vi "WLAN_FrameSync - Optimized.vi"(11 "input cluster":cluster{"t0":dbl, "dt":dbl, "Y":cdb[]}) -> (2 "is valid packet?":bool, 3 "output cluster":cluster{"t0":dbl, "dt":dbl, "Y":cdb[]})   [LabVIEW 2022 SP3]
uses:
  <vilib>/Analysis/2dsp.llb/1D Cross Correlation (CDB).vi
  <vilib>/Analysis/NI_AALPro.lvlib
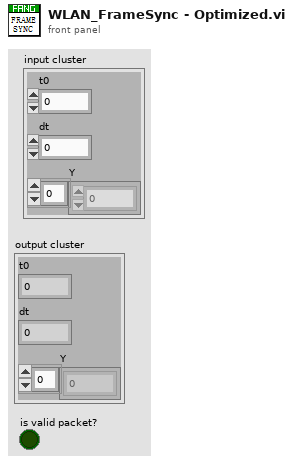
[diagram p1: front panel]
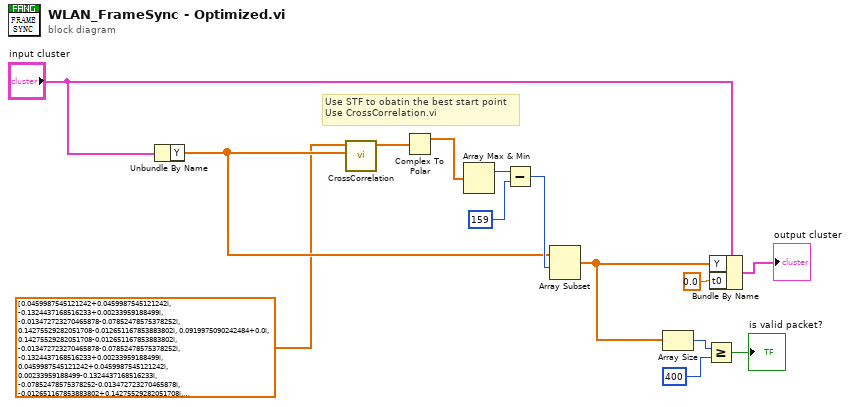
[diagram p0: block diagram]
diagram:
  # "Use STF to obatin the best start point\nUse CrossCorrelation.vi"
  n1 = Unbundle By Name("input cluster") -> ("Y"=w2:cdb[])
  n2 = call-poly <vilib>:"CrossCorrelation.vi"("Y"=w2, "X"=cdb[] [0.0459987545121242+0.0459987545121242i, -0.1324437168516233+0.00233959188499i, -0.013472723270465878-0.07852478575378252i, 0.14275529282051708-0.012651167853883802i, 0.0919975090242484+0.0i, 0.14275529282051708-0.012651167853883802i, -0.013472723270465878-0.07852478575378252i, -0.1324437168516233+0.00233959188499i, 0.0459987545121242+0.0459987545121242i, 0.00233959188499-0.1324437168516233i, -0.07852478575378252-0.013472723270465878i, -0.012651167853883802+0.14275529282051708i, 0.0+0.0919975090242484i, -0.012651167853883802+0.14275529282051708i, -0.07852478575378252-0.013472723270465878i, 0.00233959188499-0.1324437168516233i, 0.0459987545121242+0.0459987545121242i, -0.1324437168516233+0.00233959188499i, -0.013472723270465878-0.07852478575378252i, 0.14275529282051708-0.012651167853883802i, 0.0919975090242484+0.0i, 0.14275529282051708-0.012651167853883802i, -0.013472723270465878-0.07852478575378252i, -0.1324437168516233+0.00233959188499i, 0.0459987545121242+0.0459987545121242i, 0.00233959188499-0.1324437168516233i, -0.07852478575378252-0.013472723270465878i, -0.012651167853883802+0.14275529282051708i, 0.0+0.0919975090242484i, -0.012651167853883802+0.14275529282051708i, -0.07852478575378252-0.013472723270465878i, 0.00233959188499-0.1324437168516233i, 0.0459987545121242+0.0459987545121242i, -0.1324437168516233+0.00233959188499i, -0.013472723270465878-0.07852478575378252i, 0.14275529282051708-0.012651167853883802i, 0.0919975090242484+0.0i, 0.14275529282051708-0.012651167853883802i, -0.013472723270465878-0.07852478575378252i, -0.1324437168516233+0.00233959188499i, 0.0459987545121242+0.0459987545121242i, 0.00233959188499-0.1324437168516233i, -0.07852478575378252-0.013472723270465878i, -0.012651167853883802+0.14275529282051708i, 0.0+0.0919975090242484i, -0.012651167853883802+0.14275529282051708i, -0.07852478575378252-0.013472723270465878i, 0.00233959188499-0.1324437168516233i, 0.0459987545121242+0.0459987545121242i, -0.1324437168516233+0.00233959188499i, -0.013472723270465878-0.07852478575378252i, 0.14275529282051708-0.012651167853883802i, 0.0919975090242484+0.0i, 0.14275529282051708-0.012651167853883802i, -0.013472723270465878-0.07852478575378252i, -0.1324437168516233+0.00233959188499i, 0.0459987545121242+0.0459987545121242i, 0.00233959188499-0.1324437168516233i, -0.07852478575378252-0.013472723270465878i, -0.012651167853883802+0.14275529282051708i, 0.0+0.0919975090242484i, -0.012651167853883802+0.14275529282051708i, -0.07852478575378252-0.013472723270465878i, 0.00233959188499-0.1324437168516233i, 0.0459987545121242+0.0459987545121242i, -0.1324437168516233+0.00233959188499i, -0.013472723270465878-0.07852478575378252i, 0.14275529282051708-0.012651167853883802i, 0.0919975090242484+0.0i, 0.14275529282051708-0.012651167853883802i, -0.013472723270465878-0.07852478575378252i, -0.1324437168516233+0.00233959188499i, 0.0459987545121242+0.0459987545121242i, 0.00233959188499-0.1324437168516233i, -0.07852478575378252-0.013472723270465878i, -0.012651167853883802+0.14275529282051708i, 0.0+0.0919975090242484i, -0.012651167853883802+0.14275529282051708i, -0.07852478575378252-0.013472723270465878i, 0.00233959188499-0.1324437168516233i, 0.0459987545121242+0.0459987545121242i, -0.1324437168516233+0.00233959188499i, -0.013472723270465878-0.07852478575378252i, 0.14275529282051708-0.012651167853883802i, 0.0919975090242484+0.0i, 0.14275529282051708-0.012651167853883802i, -0.013472723270465878-0.07852478575378252i, -0.1324437168516233+0.00233959188499i, 0.0459987545121242+0.0459987545121242i, 0.00233959188499-0.1324437168516233i, -0.07852478575378252-0.013472723270465878i, -0.012651167853883802+0.14275529282051708i, 0.0+0.0919975090242484i, -0.012651167853883802+0.14275529282051708i, -0.07852478575378252-0.013472723270465878i, 0.00233959188499-0.1324437168516233i, 0.0459987545121242+0.0459987545121242i, -0.1324437168516233+0.00233959188499i, -0.013472723270465878-0.07852478575378252i, 0.14275529282051708-0.012651167853883802i, 0.0919975090242484+0.0i, 0.14275529282051708-0.012651167853883802i, -0.013472723270465878-0.07852478575378252i, -0.1324437168516233+0.00233959188499i, 0.0459987545121242+0.0459987545121242i, 0.00233959188499-0.1324437168516233i, -0.07852478575378252-0.013472723270465878i, -0.012651167853883802+0.14275529282051708i, 0.0+0.0919975090242484i, -0.012651167853883802+0.14275529282051708i, -0.07852478575378252-0.013472723270465878i, 0.00233959188499-0.1324437168516233i, 0.0459987545121242+0.0459987545121242i, -0.1324437168516233+0.00233959188499i, -0.013472723270465878-0.07852478575378252i, 0.14275529282051708-0.012651167853883802i, 0.0919975090242484+0.0i, 0.14275529282051708-0.012651167853883802i, -0.013472723270465878-0.07852478575378252i, -0.1324437168516233+0.00233959188499i, 0.0459987545121242+0.0459987545121242i, 0.00233959188499-0.1324437168516233i, -0.07852478575378252-0.013472723270465878i, -0.012651167853883802+0.14275529282051708i, 0.0+0.0919975090242484i, -0.012651167853883802+0.14275529282051708i, -0.07852478575378252-0.013472723270465878i, 0.00233959188499-0.1324437168516233i, 0.0459987545121242+0.0459987545121242i, -0.1324437168516233+0.00233959188499i, -0.013472723270465878-0.07852478575378252i, 0.14275529282051708-0.012651167853883802i, 0.0919975090242484+0.0i, 0.14275529282051708-0.012651167853883802i, -0.013472723270465878-0.07852478575378252i, -0.1324437168516233+0.00233959188499i, 0.0459987545121242+0.0459987545121242i, 0.00233959188499-0.1324437168516233i, -0.07852478575378252-0.013472723270465878i, -0.012651167853883802+0.14275529282051708i, 0.0+0.0919975090242484i, -0.012651167853883802+0.14275529282051708i, -0.07852478575378252-0.013472723270465878i, 0.00233959188499-0.1324437168516233i, 0.0459987545121242+0.0459987545121242i, -0.1324437168516233+0.00233959188499i, -0.013472723270465878-0.07852478575378252i, 0.14275529282051708-0.012651167853883802i, 0.0919975090242484+0.0i, 0.14275529282051708-0.012651167853883802i, -0.013472723270465878-0.07852478575378252i, -0.1324437168516233+0.00233959188499i, 0.0459987545121242+0.0459987545121242i, 0.00233959188499-0.1324437168516233i, -0.07852478575378252-0.013472723270465878i, -0.012651167853883802+0.14275529282051708i, 0.0+0.0919975090242484i, -0.012651167853883802+0.14275529282051708i, -0.07852478575378252-0.013472723270465878i, 0.00233959188499-0.1324437168516233i] ("STF")) -> ("Rxy"=w4:cdb[])  [unwired: 8 in, 1 out]
  n3 = Complex To Polar(r * e^(i*theta)=w4) -> (r=w14:dbl[])  [unwired: 1 out]
  n4 = Array Max & Min(array=w14) -> (max index (indices)=w12:i32)  [unwired: 3 out]
  n5 = Subtract(x=w12, y=159) -> (x-y=w3:i32)
  n6 = Array Subset(array=w2, index=w3) -> (w5:cdb[])  [unwired: 1 in]
  n7 = Array Size(array=w5) -> (size(s)=w8:i32)
  n8 = Greater Or Equal?(x=w8, y=400) -> (x >= y?=→"is valid packet?":bool)
  n9 = Bundle By Name(cluster="input cluster", "Y"=w5, "t0"=0.0) -> (→"output cluster":cluster{"t0":dbl, "dt":dbl, "Y":cdb[]})
